vi "Parse Node - Specific.vi"(7 "Parent ID":string, 8 "error in (no error)":errorcluster, 10 "Node in":refnum<k20>, 11 "Tree in":refnum<data-value>) -> (0 "error out":errorcluster, 2 "Node out":refnum<k20>, 3 "Tree out":refnum<data-value>, 5 "Unique ID":string)   [LabVIEW 2016]
uses:
  <vilib>/ni/Tree/Tree Manager/Tree.lvclass
  <vilib>/ni/Tree/Tree Manager/API/Set Meta Data.vi
  <resource>/objmgr/DOMUserDefRef.rc
  <vilib>/xml/NI_XML.lvlib
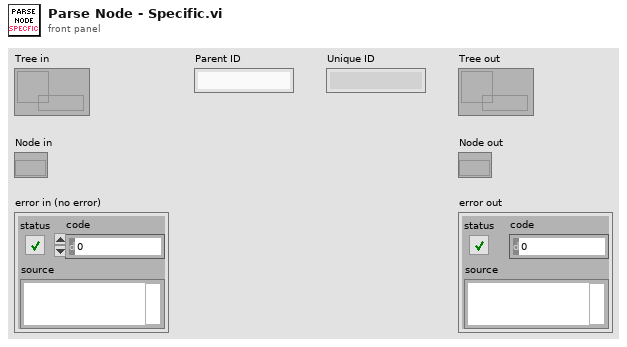
[diagram p1: front panel]
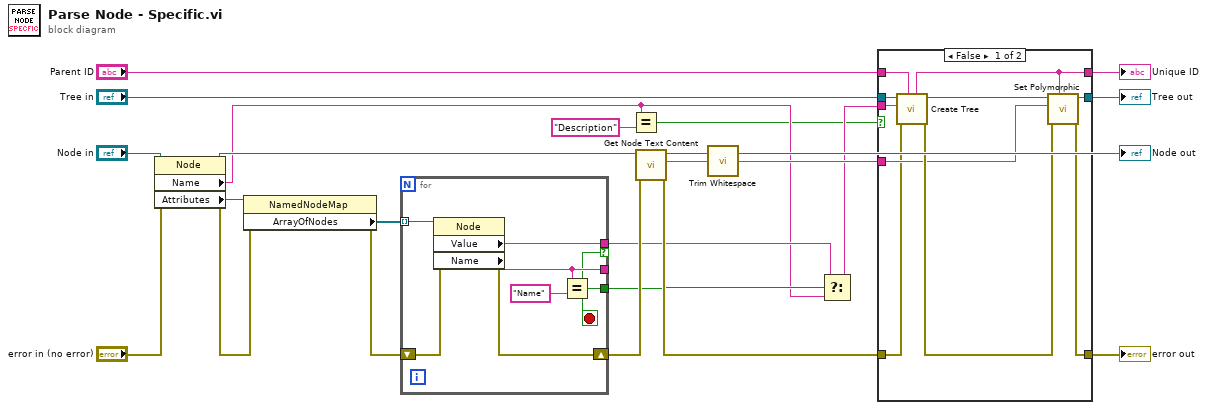
[diagram p0: block diagram]
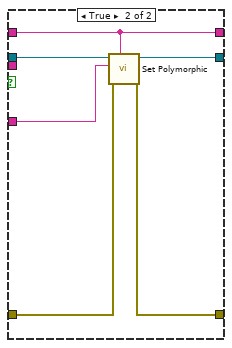
[diagram p2: hidden frame]
diagram:
  n1 = property class="Node"(reference="Node in", error in="error in (no error)") -> (reference out=w14:refnum<k20>, error out=w22:errorcluster, "Name"=w4:string, "Attributes"=w11:refnum<k20>)
  n2 = property class="NamedNodeMap"(reference=w11, error in=w22) -> (error out=w23:errorcluster, "ArrayOfNodes"=w12:refnum<k20>[])  [unwired: 1 out]
  n3 = for {
    tunnel: w12 -> [w28] mode=indexing
    shift-right: [w29] -> w19
    shift-left: w23 -> [w30]
    tunnel: [w27] -> w6 if=w24
    tunnel: [w26] -> _
    tunnel: [w24] -> w7
    stop <- w24 stop-if-true
    n4 = property class="Node"(reference=w28, error in=w30) -> (error out=w29:errorcluster, "Value"=w27:string, "Name"=w26:string)  [unwired: 1 out]
    n5 = Equal?(x=w26, y="Name") -> (x = y?=w24:bool)
  }
  n6 = Equal?(x=w4, y="Description") -> (x = y?=w1:bool)
  n7 = call <vilib>:"Get Node Text Content.vi"("error in (no error)"=w19, "node in"=w14) -> ("error out"=w20:errorcluster, "node text"=w18:string, "node out"=→"Node out":refnum<k20>)  [unwired: 7 in]
  n8 = call <vilib>:"Trim Whitespace.vi"("string"=w18) -> ("trimmed string"=w9:string)  [unwired: 1 in]
  n9 = Select(t=w6, s=w7, f=w4) -> (s? t:f=w5:string)
  n10 = case shown="False" w1 {
    tunnel: w20 -> [w32 w42]
    tunnel: [w39 w46] -> w17
    tunnel: "Parent ID" -> [w38 w46]
    tunnel: "Tree in" -> [w36 w44]
    tunnel: w9 -> [w35 w43]
    tunnel: [w34 w45] -> w8
    tunnel: w5 -> [w33 _]
    tunnel: [w31 w41] -> w2
    frame False {
      n11 = call <vilib>:"Create Tree.vi"("Parent ID (empty)"=w38, "Error In"=w32, "Name"=w33, "Tree Manager"=w36) -> ("Error Out"=w40:errorcluster, "Tree Manager"=w37:refnum<data-value>, "Unique ID"=w39:string)  [unwired: 5 in]
      n12 = call-poly <vilib>:"Set Polymorphic.vi"("Tree ID"=w39, "Error In"=w40, "Meta Data"=w35, "Tree Manager"=w37) -> ("Error Out"=w31:errorcluster, "Tree Manager"=w34:refnum<data-value>)  [unwired: 6 in]
    }
    frame True {
      n13 = call-poly <vilib>:"Set Polymorphic.vi"("Tree ID"=w46, "Error In"=w42, "Meta Data"=w43, "Tree Manager"=w44) -> ("Error Out"=w41:errorcluster, "Tree Manager"=w45:refnum<data-value>)  [unwired: 6 in]
    }
  }
  "Unique ID" <- w17
  "Tree out" <- w8
  "error out" <- w2
